vi "Dereference libssh2_knownhost.vi"(8 "error in (no error)":errorcluster, 11 "p":u64) -> (0 "error out":errorcluster, 3 "libssh2_knownhost":T1)   [LabVIEW 2013, in "libssh2.lvlib"]
uses:
  libssh2.lvlib
  libssh2_knownhost.ctl
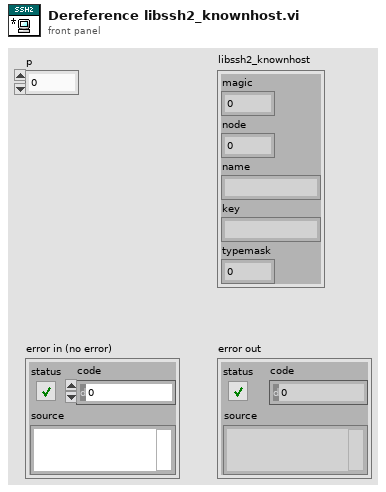
[diagram p1: front panel]
types:
  T1 = typedef "libssh2.lvlib/libssh2_knownhost.ctl" = cluster{"magic":u32, "node":u64, "name":string, "key":string, "typemask":i32}
  T2 = cluster{"magic":u32, "node":u64, "name":u64, "key":u64, "typemask":i32}
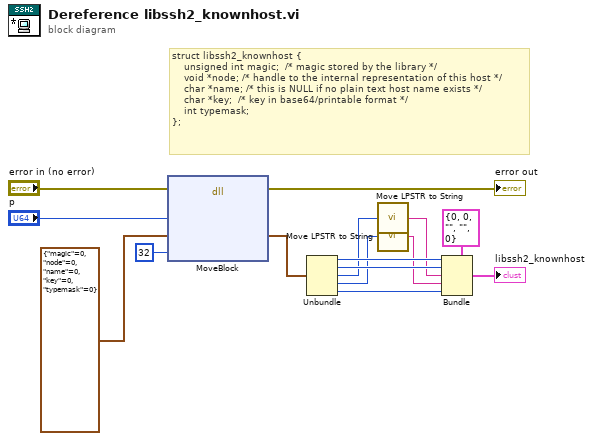
[diagram p0: block diagram]
diagram:
  # "struct libssh2_knownhost {\n    unsigned int magic;  /* magic stored by the library */\n    void *node; /* handle to the internal representation of this host */\n    char *name; /* this is NULL if no plain text host name exists */\n    char *key;  /* key in base64/printable format */\n    int typemask;\n};"
  n1 = dll-call lib="LabVIEW" fn="MoveBlock"(error in="error in (no error)", "ps"="p", "pd"=T2 {"magic"=0, "node"=0, "name"=0, "key"=0, "typemask"=0}, "size"=i64 32) -> (error out=→"error out":errorcluster, "pd"=w13:T2)  [unwired: 5 in, 1 out]
  n2 = Unbundle(w13) -> ("magic"=w12:u32, "node"=w11:u64, "name"=w5:u64, "key"=w6:u64, "typemask"=w10:i32)
  n3 = call "Move LPSTR to String.vi"("LPSTR"=w5) -> ("String"=w9:string)  [unwired: 1 in]
  n4 = call "Move LPSTR to String.vi"("LPSTR"=w6) -> ("String"=w8:string)  [unwired: 1 in]
  n5 = Bundle(cluster=T1 {"magic"=0, "node"=0, "name"="", "key"="", "typemask"=0} ("libssh2_knownhost"), "magic"=w12, "node"=w11, "name"=w9, "key"=w8, "typemask"=w10) -> (→"libssh2_knownhost":T1)
